vi "Generate User Service.vi"(7 "RPC Method Parameters":T1[](array[typedef]), 8 "error in (no error)":errorcluster, 9 ">>Application instance>> in":refnum<vi>, 10 "Service base class in":refnum<vi>, 11 "UserCode Lib in":refnum<vi>) -> (0 "error out":errorcluster, 1 ">>Application instance>> out":refnum<vi>, 2 "Service Impl class out":refnum<vi>, 3 "Service Base class out":refnum<vi>)   [LabVIEW 2019, in "gRPC Template Creation Utility.lvlib"]
uses:
  gRPC Template Creation Utility.lvlib
  TypeDefs/RPC Method Parameters.ctl
panel:
  out "UserCode Lib out":refnum<vi>
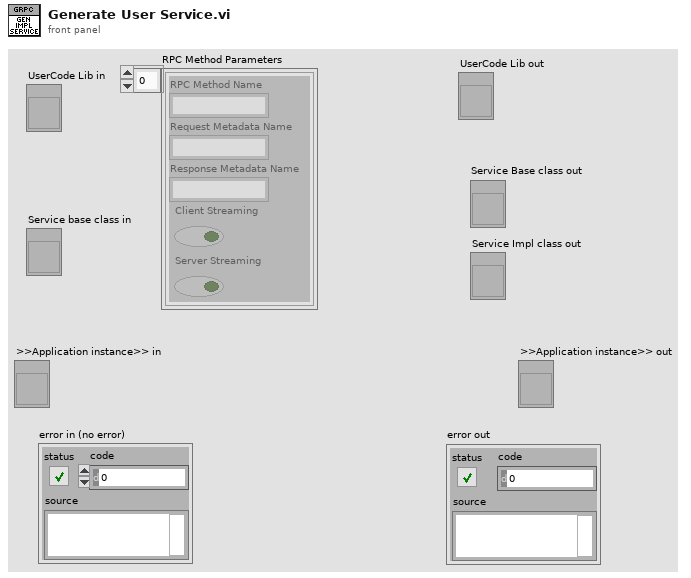
[diagram p1: front panel]
types:
  T1 = typedef "gRPC Template Creation Utility.lvlib/RPC Method Parameters.ctl" = cluster{"RPC Method Name":string, "Request Metadata Name":string, "Response Metadata Name":string, "Client Streaming":bool, "Server Streaming":bool}
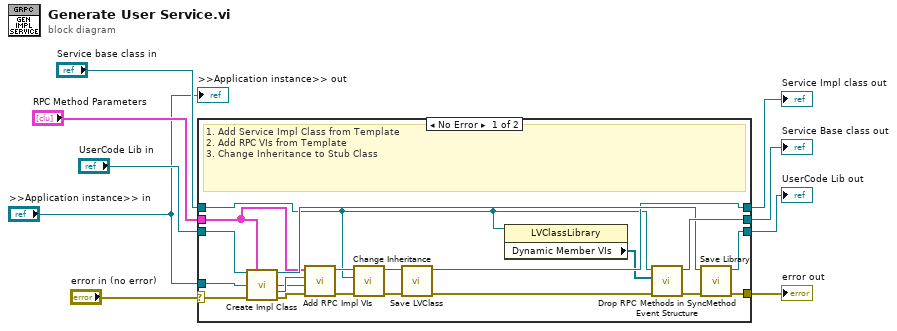
[diagram p0: block diagram]
diagram:
  n1 = case shown="No Error" "error in (no error)" {
    selector: "error in (no error)" -> [w23 w32]
    tunnel: [w25 w32] -> w8
    tunnel: "Service base class in" -> [w11 w31]
    tunnel: [w27 w31] -> w6
    tunnel: "RPC Method Parameters" -> [w12 _]
    tunnel: "UserCode Lib in" -> [w22 w30]
    tunnel: [w21 w30] -> w3
    tunnel: [w14 _] -> w2
    tunnel: ">>Application instance>> in" -> [w20 _]
    frame No Error {
      # "1. Add Service Impl Class from Template\n2. Add RPC VIs from Template\n3. Change Inheritance to Stub Class"
      n2 = call "Create Impl Class.vi"("User Server Library in"=w22, "RPC Method Parameters"=w12, ">>Application instance>> in"=w20, "error in (no error)"=w23) -> ("User Server Library out"=w24:refnum<vi>, ">>Application instance>> out"=w19:refnum<vi>, "Service Impl class out"=w29:refnum<vi>, "error IO"=w28:errorcluster)  [unwired: 8 in]
      n3 = call "Add RPC Impl VIs.vi"("error in"=w28, "Application reference in"=w19, "Service Impl class in"=w29, "RPC Method Parameters"=w12) -> ("error out"=w17:errorcluster, "Service Impl class out"=w18:refnum<vi>)  [unwired: 6 in]
      n4 = call "Change Inheritance.vi"("error in (no error)"=w17, "Parent Class"=w11, "LV Class Ref in"=w18) -> ("error out"=w15:errorcluster, "LV Class ref out"=w16:refnum<vi>)  [unwired: 7 in]
      n5 = call "Save LVClass.vi"("error in (no error)"=w15, "LVClassLibrary in"=w16) -> ("error out"=w13:errorcluster, "LVClassLibrary out"=w14:refnum<vi>)  [unwired: 8 in]
      n6 = property class="LVClassLibrary"(reference=w11) -> ("Dynamic Member VIs"=w10:refnum<vi>[])  [unwired: 1 in, 2 out]
      n7 = call "Drop RPC Methods in SyncMethod Event Structure.vi"("error in (no error)"=w13, "dynamic member VIs"=w10, "Server class in"=w11) -> ("error out"=w26:errorcluster, "Server class out"=w27:refnum<vi>)  [unwired: 7 in]
      n8 = call "Save Library.vi"("error in (no error)"=w26, "Library in"=w24) -> ("error out"=w25:errorcluster, "Library out"=w21:refnum<vi>)  [unwired: 8 in]
    }
    frame Error {
    }
  }
  "error out" <- w8
  "Service Base class out" <- w6
  "UserCode Lib out" <- w3
  "Service Impl class out" <- w2
  ">>Application instance>> out" <- ">>Application instance>> in"
